vi "OmniDriveBegin.vi"(8 "error in":errorcluster) -> (0 "error out":errorcluster)   [LabVIEW 2014]
uses:
  <vilib>/Rock Robotics/SystemInterfaces/DIO/FPGA_DIOPWMChannel.ctl
  <vilib>/Rock Robotics/WPI/SafetyOutput/WPI_SafetyOutputConfigMenu.ctl
  <vilib>/Rock Robotics/WPI/RobotDrive/WPI_RobotDriveOpen2MotorWithCANJaguar.vi
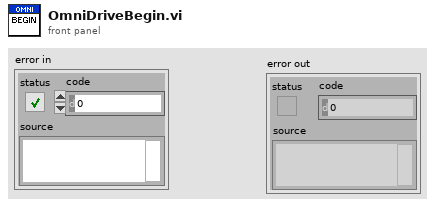
[diagram p1: front panel]
types:
  T1 = typedef "WPI_SafetyOutputConfigMenu.ctl" = enum16{"Enable", "Disable"}
  T2 = typedef "FPGA_DIOPWMChannel.ctl" = enum8{"PWM 0", "PWM 1", "PWM 2", "PWM 3", "PWM 4", "PWM 5", "PWM 6", "PWM 7", "PWM 8", "PWM 9", "PWM MXP 0", "PWM MXP 1", "PWM MXP 2", "PWM MXP 3", "PWM MXP 4", "PWM MXP 5", "PWM MXP 6", "PWM MXP 7", "PWM MXP 8", "PWM MXP 9", "Invalid"}
  T3 = typedef "WPI_RobotDriveDevRef.ctl" = cluster{"DevStatus":errorcluster, "Motors[]":T4[], "Square Inputs":bool, "Max Output":dbl}
  T4 = typedef "WPI_MotorControlDeviceRef.ctl" = cluster{"DeviceStatus":errorcluster, "Type":T5, "PWM":cluster{"Controller":T6, "PWM Channel":T2, "DeadBand":T7}, "CAN":cluster{"Device Number":u8, "Control Mode":T8, "Semaphore":T9, "Max Vout":dbl, "TalonSRX Control Mode":T10}, "Invert":bool, "TransformRef":T11, "InvTransformRef":T11}
  T5 = typedef "WPI_MotorControlType.ctl" = enum16{"PWM", "CAN", "CANTalonSRX"}
  T6 = typedef "FPGA_TypedefDigitalModule.ctl" = enum16{"Controller 1"}
  T7 = typedef "WPI_PWMDeadband.ctl" = cluster{"Name":string, "maxPositivePwm":i32, "minPositivePwm":i32, "centerPwm":i32, "maxNegativePwm":i32, "minNegativePwm":i32, "angularRange":u16}
  T8 = typedef "WPI_CANJaguar_ControlMode.ctl" = enum8{"Percent VBus", "Current", "Speed", "Position", "Voltage"}
  T9 = typedef "Semaphore RefNum" = refnum<k1>
  T10 = typedef "WPI_CANTalonSRX_APIControlMode.ctl" = enum8{"Percent VBus", "Speed", "Position", "Slave", "Unchanged / Invalid"}
  T11 = typedef "WPI_PWMTransform_ConPane.ctl" = refnum<vi>
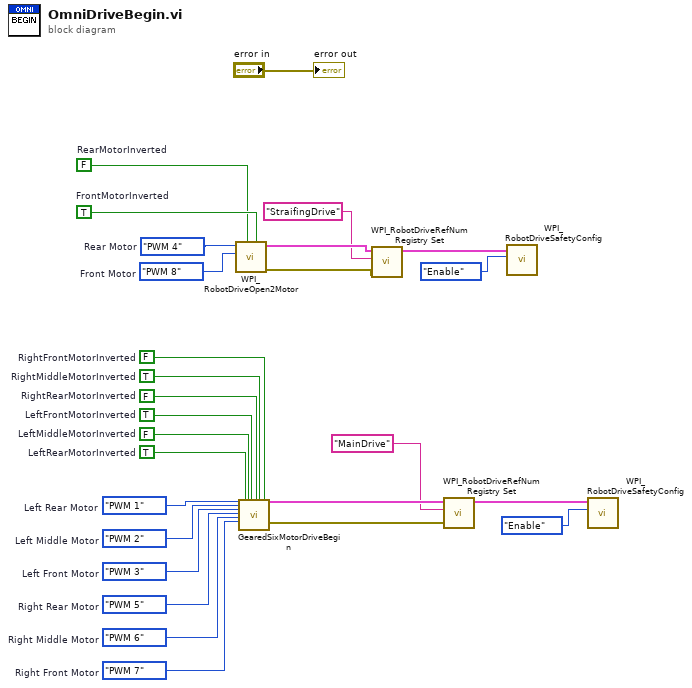
[diagram p0: block diagram]
diagram:
  w7 = FALSE  # RightRearMotorInverted
  w8 = TRUE  # RightMiddleMotorInverted
  w9 = FALSE  # RightFrontMotorInverted
  w6 = TRUE  # LeftFrontMotorInverted
  w5 = FALSE  # LeftMiddleMotorInverted
  w4 = TRUE  # LeftRearMotorInverted
  w11 = FPGA_DIOPWMChannel."PWM 7"  # Right Front Motor
  w12 = FPGA_DIOPWMChannel."PWM 6"  # Right Middle Motor
  w13 = FPGA_DIOPWMChannel."PWM 5"  # Right Rear Motor
  w14 = FPGA_DIOPWMChannel."PWM 3"  # Left Front Motor
  w15 = FPGA_DIOPWMChannel."PWM 2"  # Left Middle Motor
  w16 = FPGA_DIOPWMChannel."PWM 1"  # Left Rear Motor
  w23 = FPGA_DIOPWMChannel."PWM 4"  # Rear Motor
  w24 = FPGA_DIOPWMChannel."PWM 8"  # Front Motor
  w25 = TRUE  # FrontMotorInverted
  w10 = FALSE  # RearMotorInverted
  n1 = call-poly <vilib>:"WPI_RobotDriveOpen2Motor.vi"("Right Motor Inverted"=w25, "Left Motor Inverted"=w10, "Right Motor"=w24, "Left Motor"=w23) -> ("error out"=w22:errorcluster, "RobotDriveDevRef"=w27:T3)  [unwired: 6 in]
  n2 = call "GearedSixMotorDriveBegin.vi"("Left Rear Motor"=w16, "Left Middle Motor"=w15, "Left Front Motor"=w14, "Right Rear Motor"=w13, "Right Middle Motor"=w12, "Right Front Motor"=w11, "Left Rear Motor Inverted"=w4, "Left Middle Motor Inverted"=w5, "Left Front Motor Inverted"=w6, "Right Rear Motor Inverted"=w7, "Right Middle Motor Inverted"=w8, "Right Front Motor Inverted"=w9) -> ("error out"=w18:errorcluster, "RobotDriveDevRef"=w19:T3)  [unwired: 14 in]
  n3 = call <vilib>:"WPI_RobotDriveRefNum Registry Set.vi"("error in (no error)"=w22, "refnum name"="StraifingDrive", "RobotDriveDevRef"=w27) -> ("RobotDriveDevRef"=w20:T3)  [unwired: 7 in, 1 out]
  n4 = call <vilib>:"WPI_RobotDriveRefNum Registry Set.vi"("error in (no error)"=w18, "refnum name"="MainDrive", "RobotDriveDevRef"=w19) -> ("RobotDriveDevRef"=w2:T3)  [unwired: 7 in, 1 out]
  n5 = call <vilib>:"WPI_RobotDriveSafetyConfig.vi"("mode"=WPI_SafetyOutputConfigMenu."Enable", "RobotDriveDevRef"=w20) -> ()  [unwired: 8 in, 2 out]
  n6 = call <vilib>:"WPI_RobotDriveSafetyConfig.vi"("mode"=WPI_SafetyOutputConfigMenu."Enable", "RobotDriveDevRef"=w2) -> ()  [unwired: 8 in, 2 out]
  "error out" <- "error in"
